vi "Create LED Names_Centauro_Dryer.vi"(11 "Error In":errorcluster) -> (4 "Names":string[](array[string]), 15 "Error Out":errorcluster)   [LabVIEW 2016]
uses:
  Centauro Washer/Product Testcode/Centauro/Valew Common/type defs/LED Status OOB.ctl
panel:
  in  "Expected LED Status":T2={"Damp"=enum."On", "Dry"=enum."Off", "Cool"=enum."Off", "Eco"=enum."Off"}
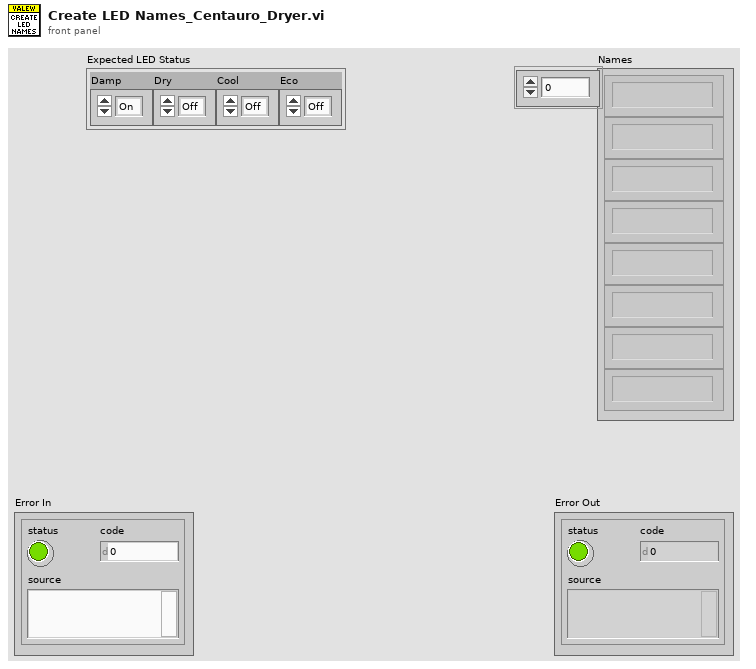
[diagram p1: front panel]
types:
  T1 = typedef "LED Status OOB.ctl" = enum32{"Off", "On", "Blink"}
  T2 = cluster{"Damp":T1, "Dry":T1, "Cool":T1, "Eco":T1}
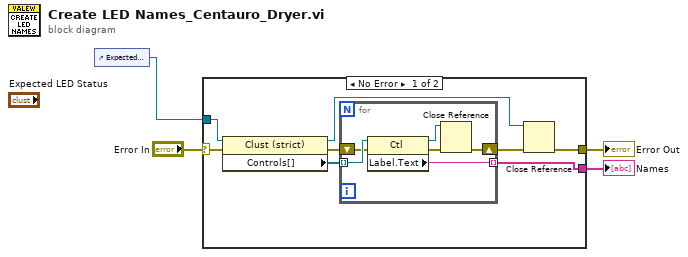
[diagram p0: block diagram]
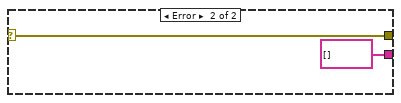
[diagram p2: hidden frame]
diagram:
  n1 = control-ref of="Expected LED Status"() -> (w1:refnum<vi>)
  n2 = case shown="No Error" "Error In" {
    selector: "Error In" -> [w7 w20]
    tunnel: [w8 w20] -> w4
    tunnel: [w6 string[] []] -> w2
    tunnel: w1 -> [w5 _]
    frame No Error {
      n3 = property class="Clust (strict)"(reference=w5, error in=w7) -> (reference out=w9:refnum<vi>, error out=w11:errorcluster, "Controls[]"=w12:refnum<vi>[])
      n4 = for {
        tunnel: w12 -> [w18] mode=indexing
        shift-right: [w14] -> w10
        shift-left: w11 -> [w17]
        tunnel: [w13] -> w6 mode=indexing
        n5 = property class="Ctl"(reference=w18, error in=w17) -> (reference out=w16:refnum<vi>, error out=w15:errorcluster, "Label.Text"=w13:string)
        n6 = Close Reference(reference=w16, error in (no error)=w15) -> (error out=w14:errorcluster)
      }
      n7 = Close Reference(reference=w9, error in (no error)=w10) -> (error out=w8:errorcluster)
    }
    frame Error {
    }
  }
  "Error Out" <- w4
  "Names" <- w2
